vi "Numeros.vi"(11 "Palabra":string) -> (1 "Boolean":bool, 2 "Numeric":u8, 3 "string":string)   [LabVIEW 2017]
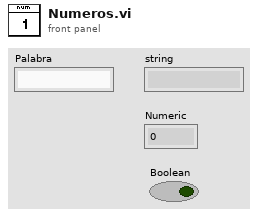
[diagram p1: front panel]
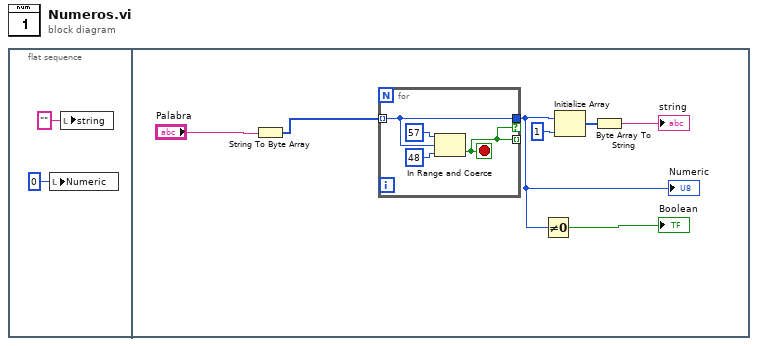
[diagram p0: block diagram]
diagram:
  n1 = flat-sequence {
    frame #0 {
      n2 = local write "Numeric"(u8 0 ("Numeric")) -> ()
      n3 = local write "string"("" ("string")) -> ()
    }
    frame #1 {
      n4 = String To Byte Array(string="Palabra") -> (unsigned byte array=w9:u8[])
      n5 = for {
        tunnel: w9 -> [w10] mode=indexing
        tunnel: [w10] -> w4 if=w11
        tunnel: [w11] -> _ mode=indexing
        stop <- w11 stop-if-true
        n6 = In Range and Coerce(upper limit=u8 57, x=w10, lower limit=u8 48) -> (In Range?=w11:bool)  [unwired: 1 out]
      }
      "Numeric" <- w4
      n7 = Not Equal To 0?(x=w4) -> (x != 0?=→"Boolean":bool)
      n8 = Initialize Array(w4, 1 ("dimension size")) -> (w5:u8[])
      n9 = Byte Array To String(unsigned byte array=w5) -> (string=→"string":string)
    }
  }
